vi "PipelineDuty.vi"(8 "error in (no error)":errorcluster, 10 "DataExchange":T1, 11 "GRMActor in":refnum<class "FlatField.lvclass">) -> (0 "error out":errorcluster, 2 "DataExchange 2":T1, 3 "GRMActor out":refnum<class "FlatField.lvclass">)   [LabVIEW 2020, in "FlatField.lvlib" / "FlatField.lvclass"]
uses:
  FlatField.lvclass
  Hardware Abstraction Layer/Component/Device/Device/DataExchange.ctl
  <vilib>/vision/Image Controls.llb/IMAQ Image.ctl
  FlatField.lvclass/FlatField.ctl
  FlatField Status.ctl
  Interface/DataListener Messages/OnDataChange Msg/OnDataChange Msg.lvclass/OnDataChange Msg.ctl
  <vilib>/ActorFramework/Message Enqueuer/Message Enqueuer.lvclass/Message Enqueuer.ctl
  <vilib>/ActorFramework/Message Enqueuer/Enqueue.vi
  Interface/DataListener Messages/OnDataChange Msg/OnDataChange Msg.lvclass
  C:/Program Files/National Instruments/LabVIEW 2020/vi.lib/ActorFramework/Message/Message.lvclass
  <vilib>/ActorFramework/Message Priority Queue/Priority Enqueue.vi
  Hardware Abstraction Layer/Component/GenericActor/GenericActor/GenericActor.lvclass
  Interface/DataListener/DataListener.lvclass
  <vilib>/vision/NI_Vision_Development_Module.lvlib
panel:
  out "Source":string
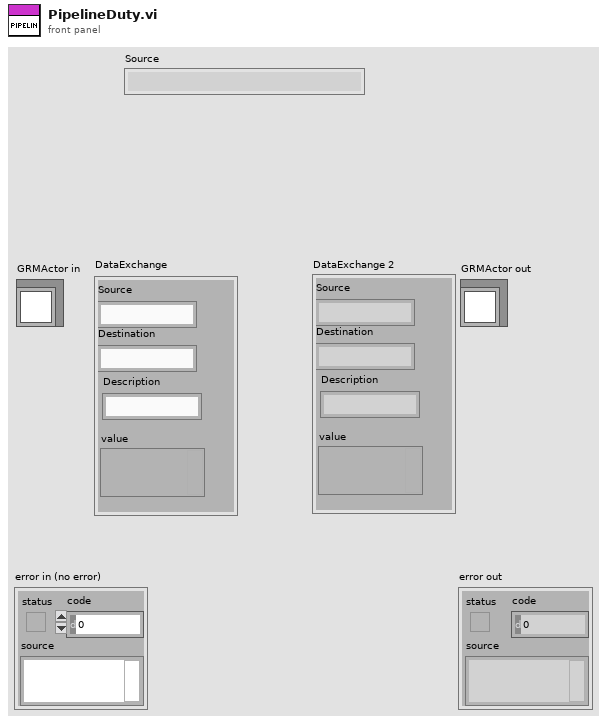
[diagram p1: front panel]
types:
  T1 = typedef "DataListener.lvclass/DataExchange.ctl" = cluster{"Source":string, "Destination":string, "Description":string, "value":variant}
  T2 = typedef "IMAQ Image.ctl" = refnum<image>
  T3 = typedef "FlatField.lvlib/FlatField.lvclass/FlatField Status.ctl" = i32
  T4 = typedef "FlatField.lvlib/FlatField.lvclass/FlatField Method.ctl" = i32
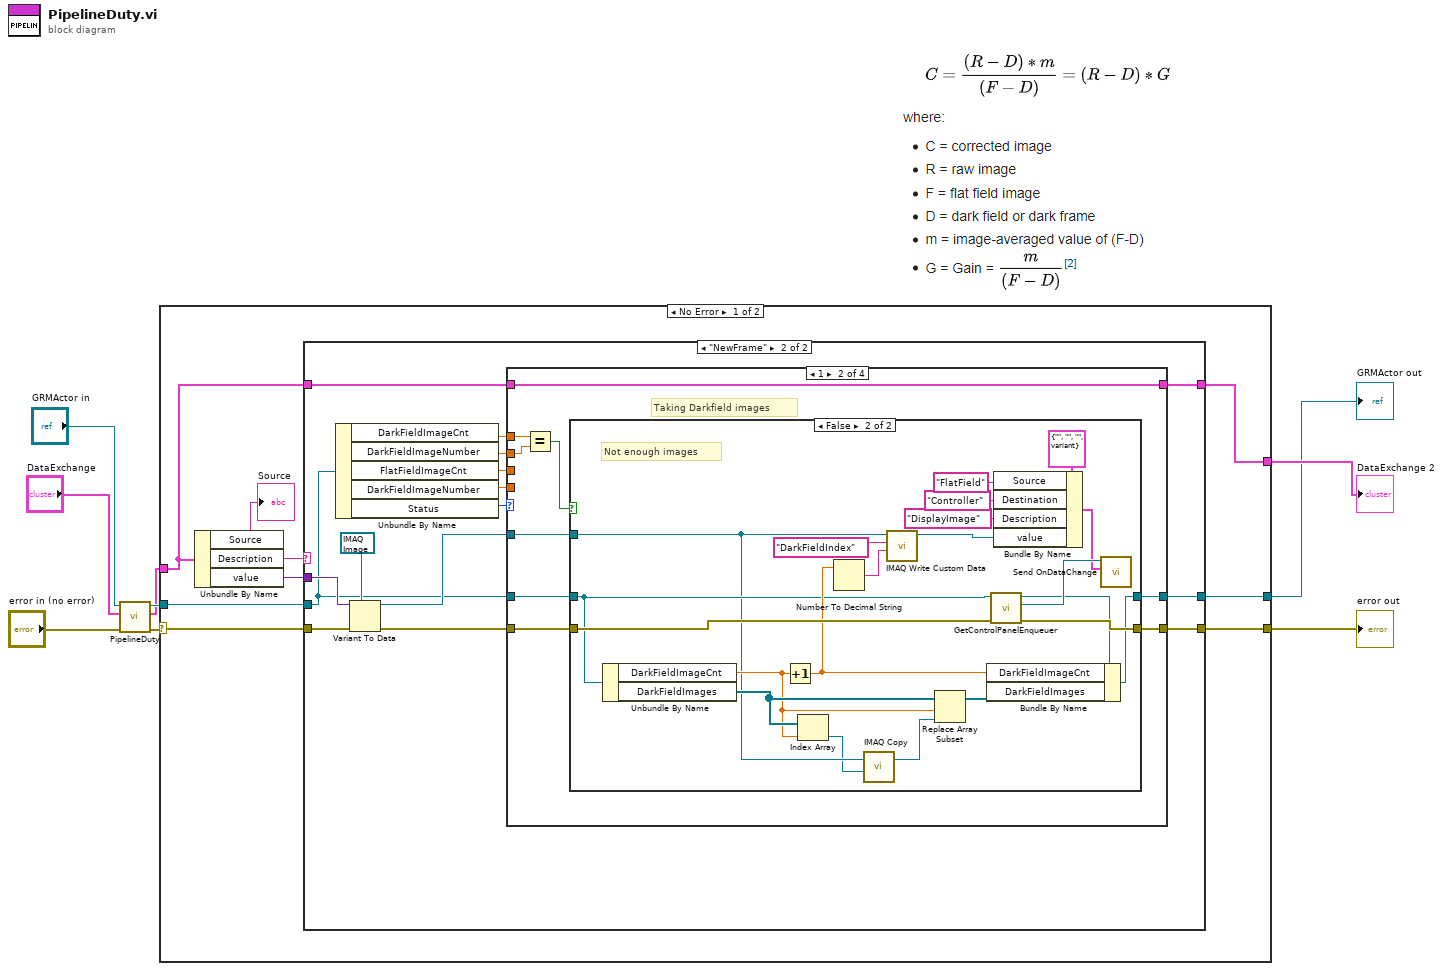
[diagram p0: block diagram]
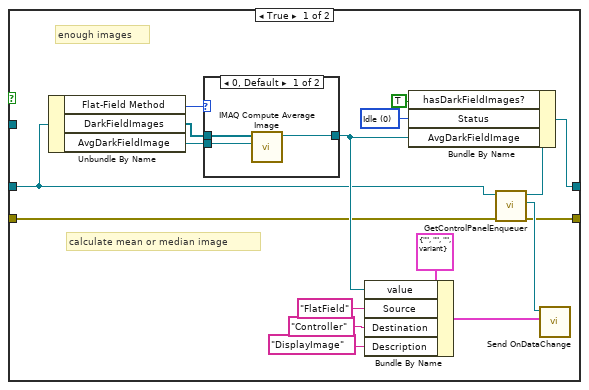
[diagram p4: hidden frame]
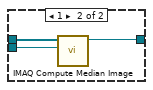
[diagram p5: hidden frame]
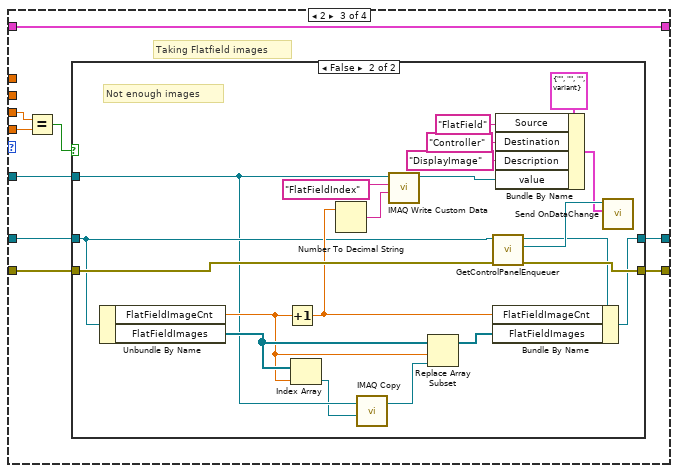
[diagram p6: hidden frame]
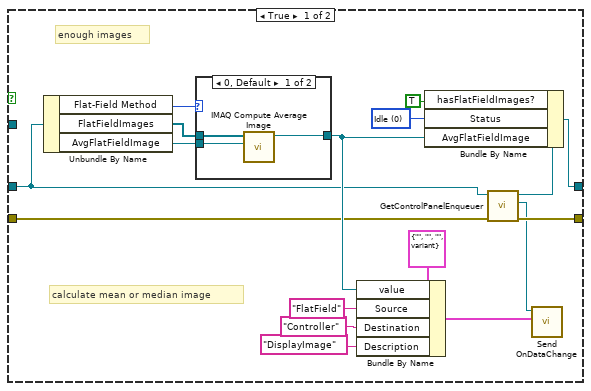
[diagram p7: hidden frame]
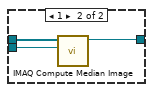
[diagram p8: hidden frame]
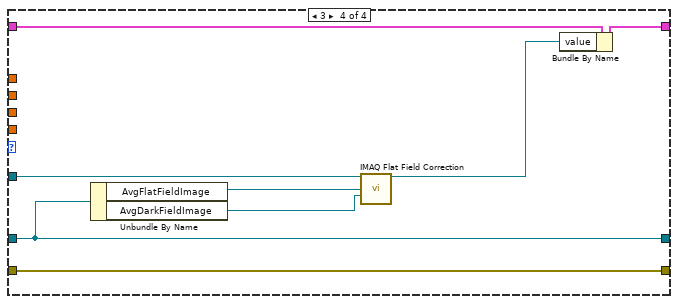
[diagram p9: hidden frame]
diagram:
  n1 = call-parent "PipelineDuty.vi"("error in (no error)"="error in (no error)", "DataExchange"="DataExchange", "GRMActor in"="GRMActor in") -> ("error out"=w6:errorcluster, "DataExchange 2"=w4:T1, "GRMActor out"=w5:refnum<class "FlatField.lvclass">)  [unwired: 6 in]
  n2 = case shown="No Error" w6 {
    selector: w6 -> [w16 w156]
    tunnel: [w17 w156] -> w1
    tunnel: w5 -> [w13 w155]
    tunnel: [w18 w155] -> w2
    tunnel: w4 -> [w12 w154]
    tunnel: [w11 w154] -> w3
    frame No Error {
      n3 = Unbundle By Name(w12) -> ("Source"=→"Source":string, "Description"=w15:string, "value"=w14:variant)
      n4 = case shown="\"NewFrame\"" w15 {
        tunnel: w14 -> [_ w35]
        tunnel: [w21 w31] -> w18
        tunnel: w13 -> [w21 w29]
        tunnel: [w20 w32] -> w17
        tunnel: w16 -> [w20 w36]
        tunnel: w12 -> [w19 w23]
        tunnel: [w19 w22] -> w11
        frame Default {
        }
        frame "NewFrame" {
          n5 = Unbundle By Name(w29) -> ("DarkFieldImageCnt"=w27:dbl, "DarkFieldImageNumber"=w26:dbl, "FlatFieldImageCnt"=w25:dbl, "DarkFieldImageNumber"=w24:dbl, "Status"=w28:T3)
          n6 = Variant To Data(error in=w36, type=T2 refnum ("New Image"), Variant=w35) -> (data=w30:T2, error out=w33:errorcluster)
          n7 = case shown="1" w28 {
            tunnel: w33 -> [w38 w48 w101 w153]
            tunnel: [w38 w47 w100 w153] -> w32
            tunnel: [w39 w46 w99 w151] -> w31
            tunnel: w30 -> [_ w44 w97 w149]
            tunnel: w29 -> [w39 w45 w98 w151]
            tunnel: w27 -> [_ w43 _ _]
            tunnel: w26 -> [_ w42 _ _]
            tunnel: w25 -> [_ _ w94 _]
            tunnel: w24 -> [_ _ w93 _]
            tunnel: w23 -> [w37 w40 w95 w152]
            tunnel: [w37 w40 w95 w150] -> w22
            frame 0, Default {
              # "idle"
            }
            frame 1 {
              # "Taking Darkfield images"
              n8 = Equal?(x=w43, y=w42) -> (x = y?=w41:bool)
              n9 = case shown="False" w41 {
                tunnel: w48 -> [w54 w92]
                tunnel: [w55 w91] -> w47
                tunnel: [w51 w78] -> w46
                tunnel: w45 -> [w53 w80]
                tunnel: w44 -> [_ w74]
                frame True {
                  w50 = T3 0 items=["Idle", "Taking DarkField Images", "Taking FlatField Image", "Doing FlatField", ""] ("Flat-Field Status")
                  # "calculate mean or median image"
                  # "enough images"
                  n10 = Unbundle By Name(w53) -> ("Flat-Field Method"=w57:T4, "DarkFieldImages"=w59:T2[], "AvgDarkFieldImage"=w58:T2)
                  n11 = case shown="0, Default" w57 {
                    tunnel: [w66 w71] -> w56
                    tunnel: w59 -> [w68 w70]
                    tunnel: w58 -> [w67 w69]
                    frame 0, Default {
                      n12 = call "IMAQ Compute Average Image"("Image Dst"=w67, "Images"=w68) -> ("Image Dst Out"=w66:T2)  [unwired: 8 in, 1 out]
                    }
                    frame 1 {
                      n13 = call "IMAQ Compute Median Image"("Image Dst"=w69, "Images"=w70) -> ("Image Dst Out"=w71:T2)  [unwired: 8 in, 1 out]
                    }
                  }
                  n14 = Bundle By Name(cluster=T1 {"Source"="", "Destination"="", "Description"="", "value"=variant} ("DataExchange"), "value"=w56, "Source"="FlatField", "Destination"="Controller", "Description"="DisplayImage") -> (w64:T1)
                  n15 = call-dynamic "GetControlPanelEnqueuer.vi"("error in (no error)"=w54, "GRMActor in"=w53) -> ("error out"=w55:errorcluster, "ControlViewEnqueuer"=w60:refnum<class "Message Enqueuer.lvclass">, "GRMActor out"=w52:refnum<class "FlatField.lvclass">)  [unwired: 7 in]
                  n16 = Bundle By Name(cluster=w52, "hasDarkFieldImages?"=TRUE, "Status"=w50, "AvgDarkFieldImage"=w56) -> (w51:refnum<class "FlatField.lvclass">)
                  n17 = call "Send OnDataChange.vi"("DataExchange"=w64, "Message Enqueuer"=w60) -> ()  [unwired: 8 in, 2 out]
                }
                frame False {
                  # "Not enough images"
                  n18 = Unbundle By Name(w80) -> ("DarkFieldImageCnt"=w75:dbl, "DarkFieldImages"=w76:T2[])
                  n19 = Increment(x=w75) -> (x+1=w81:dbl)
                  n20 = Index Array "Index Array"(array=w76, index=w75) -> (element=w73:T2)
                  n21 = Number To Decimal String(number=w81) -> (decimal integer string=w82:string)  [unwired: 1 in]
                  n22 = call "IMAQ Copy"("Image Dst"=w73, "Image Src"=w74) -> ("Image Dst Out"=w72:T2)  [unwired: 4 in, 1 out]
                  n23 = call "IMAQ Write Custom Data"("Custom Data In"=w82, "Key"="DarkFieldIndex", "Image"=w74) -> ("Image Out"=w84:T2)  [unwired: 7 in, 1 out]
                  n24 = Replace Array Subset "Replace Array Subset"(array=w76, new element=w72, index=w75) -> (w77:T2[])
                  n25 = call-dynamic "GetControlPanelEnqueuer.vi"("error in (no error)"=w92, "GRMActor in"=w80) -> ("error out"=w91:errorcluster, "ControlViewEnqueuer"=w90:refnum<class "Message Enqueuer.lvclass">, "GRMActor out"=w79:refnum<class "FlatField.lvclass">)  [unwired: 7 in]
                  n26 = Bundle By Name(cluster=w79, "DarkFieldImageCnt"=w81, "DarkFieldImages"=w77) -> (w78:refnum<class "FlatField.lvclass">)
                  n27 = Bundle By Name(cluster=T1 {"Source"="", "Destination"="", "Description"="", "value"=variant} ("DataExchange"), "Source"="FlatField", "Destination"="Controller", "Description"="DisplayImage", "value"=w84) -> (w88:T1)
                  n28 = call "Send OnDataChange.vi"("DataExchange"=w88, "Message Enqueuer"=w90) -> ()  [unwired: 8 in, 2 out]
                }
              }
            }
            frame 2 {
              # "Taking Flatfield images"
              n29 = Equal?(x=w94, y=w93) -> (x = y?=w96:bool)
              n30 = case shown="False" w96 {
                tunnel: w101 -> [w107 w145]
                tunnel: [w113 w144] -> w100
                tunnel: [w104 w131] -> w99
                tunnel: w98 -> [w106 w133]
                tunnel: w97 -> [_ w126]
                frame True {
                  w103 = T3 0 items=["Idle", "Taking DarkField Images", "Taking FlatField Image", "Doing FlatField", ""] ("Flat-Field Status")
                  # "calculate mean or median image"
                  # "enough images"
                  n31 = Unbundle By Name(w106) -> ("Flat-Field Method"=w109:T4, "FlatFieldImages"=w111:T2[], "AvgFlatFieldImage"=w110:T2)
                  n32 = case shown="0, Default" w109 {
                    tunnel: [w119 w124] -> w108
                    tunnel: w111 -> [w121 w123]
                    tunnel: w110 -> [w120 w122]
                    frame 0, Default {
                      n33 = call "IMAQ Compute Average Image"("Image Dst"=w120, "Images"=w121) -> ("Image Dst Out"=w119:T2)  [unwired: 8 in, 1 out]
                    }
                    frame 1 {
                      n34 = call "IMAQ Compute Median Image"("Image Dst"=w122, "Images"=w123) -> ("Image Dst Out"=w124:T2)  [unwired: 8 in, 1 out]
                    }
                  }
                  n35 = Bundle By Name(cluster=T1 {"Source"="", "Destination"="", "Description"="", "value"=variant} ("DataExchange"), "value"=w108, "Source"="FlatField", "Destination"="Controller", "Description"="DisplayImage") -> (w117:T1)
                  n36 = call-dynamic "GetControlPanelEnqueuer.vi"("error in (no error)"=w107, "GRMActor in"=w106) -> ("error out"=w113:errorcluster, "ControlViewEnqueuer"=w112:refnum<class "Message Enqueuer.lvclass">, "GRMActor out"=w105:refnum<class "FlatField.lvclass">)  [unwired: 7 in]
                  n37 = Bundle By Name(cluster=w105, "hasFlatFieldImages?"=TRUE, "Status"=w103, "AvgFlatFieldImage"=w108) -> (w104:refnum<class "FlatField.lvclass">)
                  n38 = call "Send OnDataChange.vi"("DataExchange"=w117, "Message Enqueuer"=w112) -> ()  [unwired: 8 in, 2 out]
                }
                frame False {
                  # "Not enough images"
                  n39 = Unbundle By Name(w133) -> ("FlatFieldImageCnt"=w127:dbl, "FlatFieldImages"=w129:T2[])
                  n40 = Increment(x=w127) -> (x+1=w134:dbl)
                  n41 = Index Array(array=w129, index=w127) -> (element=w125:T2)
                  n42 = Number To Decimal String(number=w134) -> (decimal integer string=w135:string)  [unwired: 1 in]
                  n43 = call "IMAQ Copy"("Image Dst"=w125, "Image Src"=w126) -> ("Image Dst Out"=w130:T2)  [unwired: 4 in, 1 out]
                  n44 = call "IMAQ Write Custom Data"("Custom Data In"=w135, "Key"="FlatFieldIndex", "Image"=w126) -> ("Image Out"=w137:T2)  [unwired: 7 in, 1 out]
                  n45 = Replace Array Subset "Replace Array Subset"(array=w129, new element=w130, index=w127) -> (w128:T2[])
                  n46 = call-dynamic "GetControlPanelEnqueuer.vi"("error in (no error)"=w145, "GRMActor in"=w133) -> ("error out"=w144:errorcluster, "ControlViewEnqueuer"=w143:refnum<class "Message Enqueuer.lvclass">, "GRMActor out"=w132:refnum<class "FlatField.lvclass">)  [unwired: 7 in]
                  n47 = Bundle By Name(cluster=w132, "FlatFieldImageCnt"=w134, "FlatFieldImages"=w128) -> (w131:refnum<class "FlatField.lvclass">)
                  n48 = Bundle By Name(cluster=T1 {"Source"="", "Destination"="", "Description"="", "value"=variant} ("DataExchange"), "Source"="FlatField", "Destination"="Controller", "Description"="DisplayImage", "value"=w137) -> (w141:T1)
                  n49 = call "Send OnDataChange.vi"("DataExchange"=w141, "Message Enqueuer"=w143) -> ()  [unwired: 8 in, 2 out]
                }
              }
            }
            frame 3 {
              n50 = Unbundle By Name(w151) -> ("AvgFlatFieldImage"=w148:T2, "AvgDarkFieldImage"=w147:T2)
              n51 = call "IMAQ Flat Field Correction"("Image Src"=w149, "Flat Field Image"=w148, "Dark Field Image"=w147) -> ("Corrected Image"=w146:T2)  [unwired: 10 in, 2 out]
              n52 = Bundle By Name(cluster=w152, "value"=w146) -> (w150:T1)
            }
          }
        }
      }
    }
    frame Error {
    }
  }
  "error out" <- w1
  "GRMActor out" <- w2
  "DataExchange 2" <- w3
